vi "GetTemperature.vi"(8 "error in (no error)":errorcluster, 11 "CameraSession  in":refnum<class "CS250-CameraHardwareClass.lvclass">) -> (0 "error out":errorcluster, 2 "TReading(degC/100)":i16, 3 "CameraSession out":refnum<class "CS250-CameraHardwareClass.lvclass">)   [LabVIEW 2013, in "CS250-CameraHardwareClass.lvclass"]
uses:
  CS250-CameraHardwareClass.lvclass
  CS250-CameraHardwareClass.lvclass/CS250-CameraHardwareClass.ctl
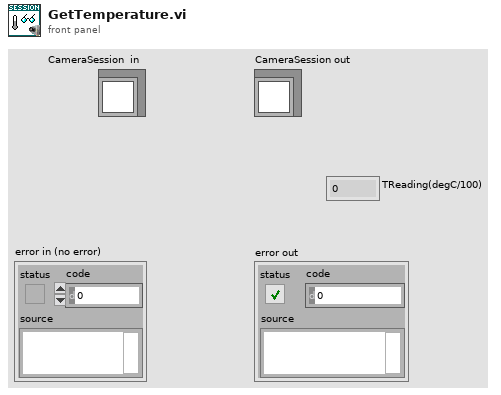
[diagram p1: front panel]
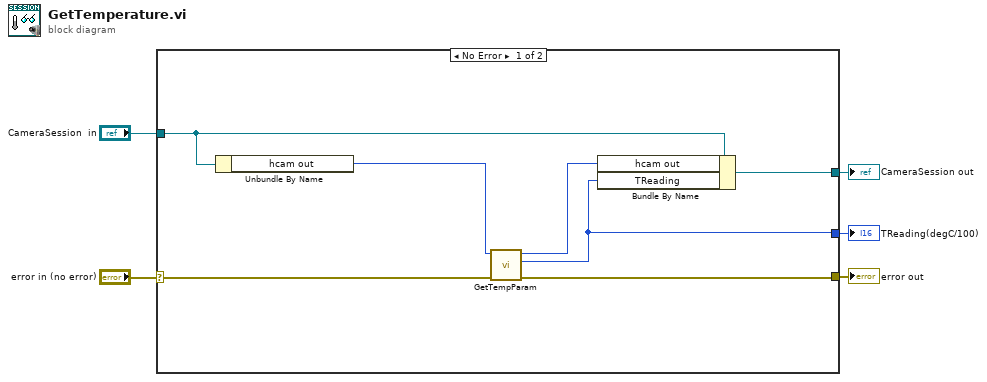
[diagram p0: block diagram]
diagram:
  n1 = case shown="No Error" "error in (no error)" {
    selector: "error in (no error)" -> [w11 w13]
    tunnel: [w7 w14] -> w4
    tunnel: "CameraSession  in" -> [w12 w14]
    tunnel: [w10 w13] -> w2
    tunnel: [w6 _] -> w1
    frame No Error {
      n2 = Unbundle By Name(w12) -> ("hcam out"=w9:i16)
      n3 = call "GetTempParam.vi"("error in (no error)"=w11, "hcam in"=w9) -> ("error out"=w10:errorcluster, "TSetpointReadback(degC/100)"=w6:i16, "hcam out"=w8:i16)  [unwired: 7 in]
      n4 = Bundle By Name(cluster=w12, "hcam out"=w8, "TReading"=w6) -> (w7:refnum<class "CS250-CameraHardwareClass.lvclass">)
    }
    frame Error {
    }
  }
  "CameraSession out" <- w4
  "error out" <- w2
  "TReading(degC/100)" <- w1
